vi "PrepareSequenceAcquisition.vi"(0 "Camera in":refnum<class "Camera.lvclass">, 11 "error in (no error)":errorcluster) -> (4 "Camera out":refnum<class "Camera.lvclass">, 6 "Setting.Exposure":i32, 8 "Setting.FramesToCapture":i32, 10 "Setting.Interval":i32, 15 "error out":errorcluster)   [LabVIEW 2020]
uses:
  Camera.lvclass
  E:/Development/DevHardSoftware/MMicroscopyAF/Model/HAL Layer/Component/Device/Device/Device.lvclass
  C:/Program Files/National Instruments/LabVIEW 2020/vi.lib/ActorFramework/Actor/Actor.lvclass
  E:/Development/DevHardSoftware/MMicroscopyAF/Model/HAL Layer/Component/Camera/Camera/Camera.lvclass
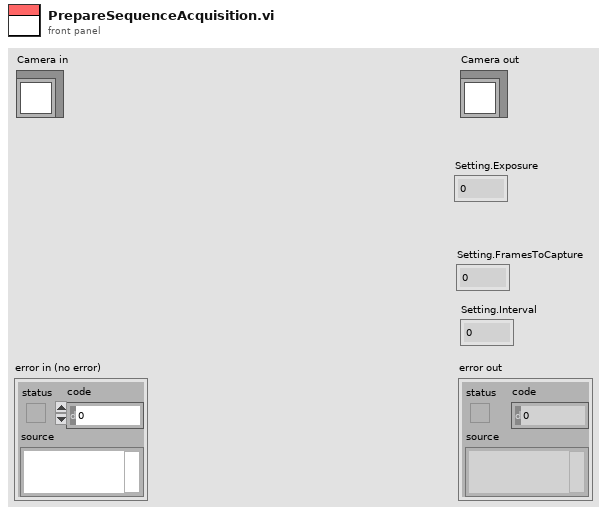
[diagram p1: front panel]
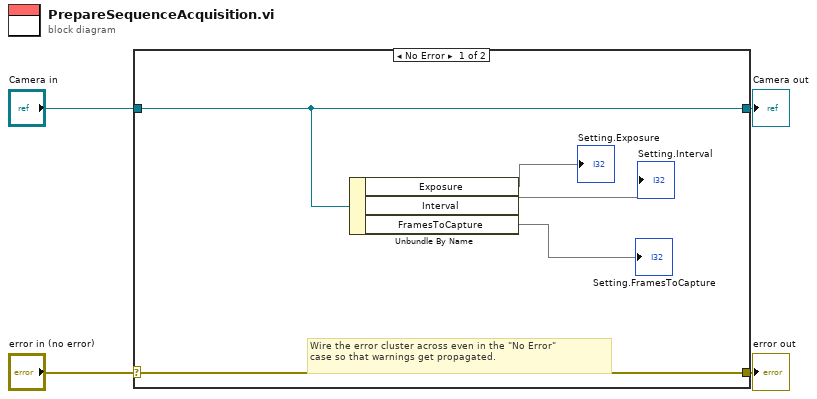
[diagram p0: block diagram]
diagram:
  n1 = case shown="No Error" "error in (no error)" {
    selector: "error in (no error)" -> [w9 w11]
    tunnel: [w9 w11] -> w3
    tunnel: [w8 w10] -> w1
    tunnel: "Camera in" -> [w8 w10]
    frame No Error {
      # "Wire the error cluster across even in the \"No Error\"\ncase so that warnings get propagated."
      n2 = Unbundle By Name(w8) -> ("Exposure"=→"Setting.Exposure", "Interval"=→"Setting.Interval", "FramesToCapture"=→"Setting.FramesToCapture")
    }
    frame Error {
    }
  }
  "error out" <- w3
  "Camera out" <- w1
